vi "Get On-Line Status.vi"(8 "error in (no error)":errorcluster, 11 "Scenarios Class in":refnum<class "Scenarios Class.lvclass">) -> (0 "error out":errorcluster, 2 "On-Line":bool, 3 "Scenarios Class out":refnum<class "Scenarios Class.lvclass">)   [LabVIEW 2020, in "SECS Scenarios.lvlib" / "Scenarios Class.lvclass"]
uses:
  Scenarios Class.lvclass
  Scenarios Class.lvclass/Scenarios Class.ctl
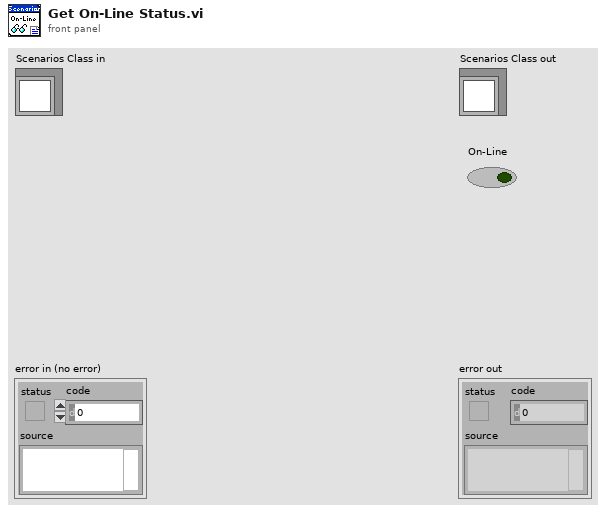
[diagram p1: front panel]
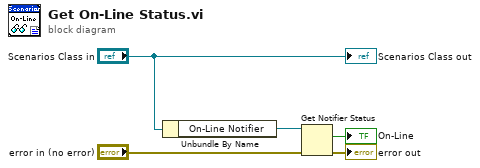
[diagram p0: block diagram]
diagram:
  n1 = Unbundle By Name("Scenarios Class in") -> ("On-Line Notifier"=w4:refnum<notifier>)
  n2 = Get Notifier Status(notifier=w4, error in (no error)="error in (no error)") -> (current notification=→"On-Line":bool, error out=→"error out":errorcluster)  [unwired: 3 out]
  "Scenarios Class out" <- "Scenarios Class in"
